vi "Sig2MS dialogPyScript.vi"(8 "error in (no error)":errorcluster) -> (0 "error out":errorcluster)   [LabVIEW 2018]
uses:
  winForms/winForms editorType.ctl
  C:/ATI_MS_InstrumentControl/dll/ScintillaNET.dll
  dll/ScintillaNET.dll
  QMH/QMH.lvclass
  Sig2MS.lvclass
  System.Windows.Forms
panel:
  in  "searchString":string
  in  "SaveScript_new":bool
  in  "open script":bool caption="OpenScript"
  in  "helper":bool caption="helpBtn"
  in  "script":refnum<k24>(container)
  in  "msgListbox":i32(listbox)
  in  "cancelBtn":bool
  in  "submitBtn":bool
  in  "stop":bool
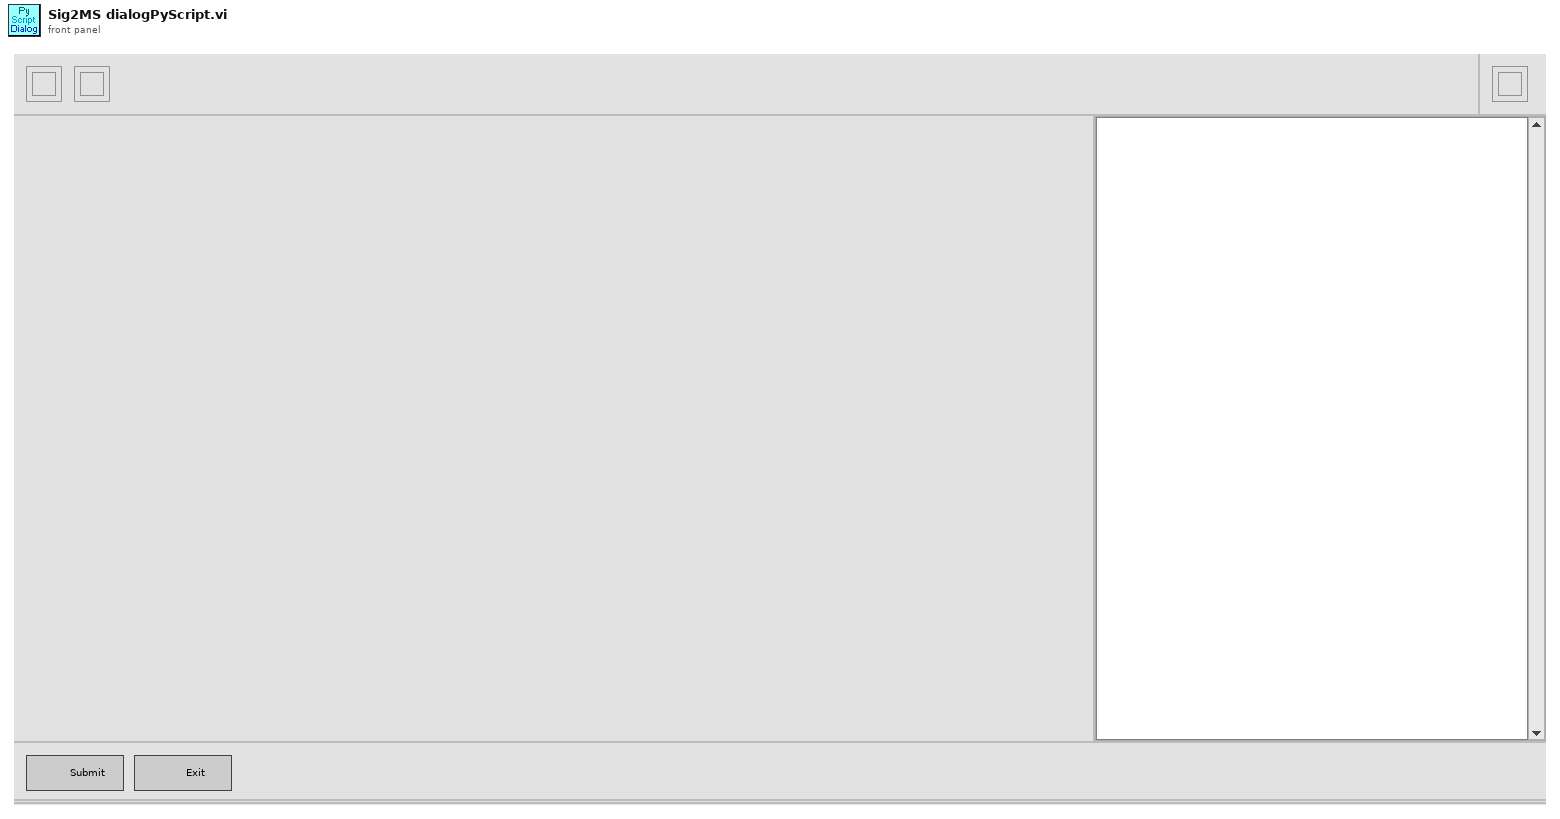
[diagram p1: front panel]
types:
  T1 = enum16{"init", "loadScript", "newScript", "runScript", "close"}
  T2 = enum8{"Enabled", "Disabled", "Disabled and Grayed Out"}
  T3 = typedef "winForms editorType.ctl" = enum16{"Recipe", "SigProc", "Editor"}
  T4 = enum16{"open", "replace", "create", "open or create", "replace or create", "replace or create with confirmation"}
  T5 = typedef "eventvkey.ctl" = enum16{"ASCII", "Enter", "Return", "Shift", "Ctrl", "Alt", "Cmd", "Opt", "Caps", "NumLock", "Clear", "Break", "Up", "Down", "Left", "Right", "Insert", "Delete", "Home", "End", "PageUp", "PageDown", "Escape", "Help", "Pause", "ScrollLock", "F1", "F2", "F3", "F4", "F5", "F6", "F7", "F8", "F9", "F10", "F11", "F12", "F13", "F14", "F15", "F16", "F17", "F18", "F19", "F20", "F21", "F22", "F23", "F24", "Play", "VolumeUp", "VolumeDown", "Mute", "Two Byte Char"}
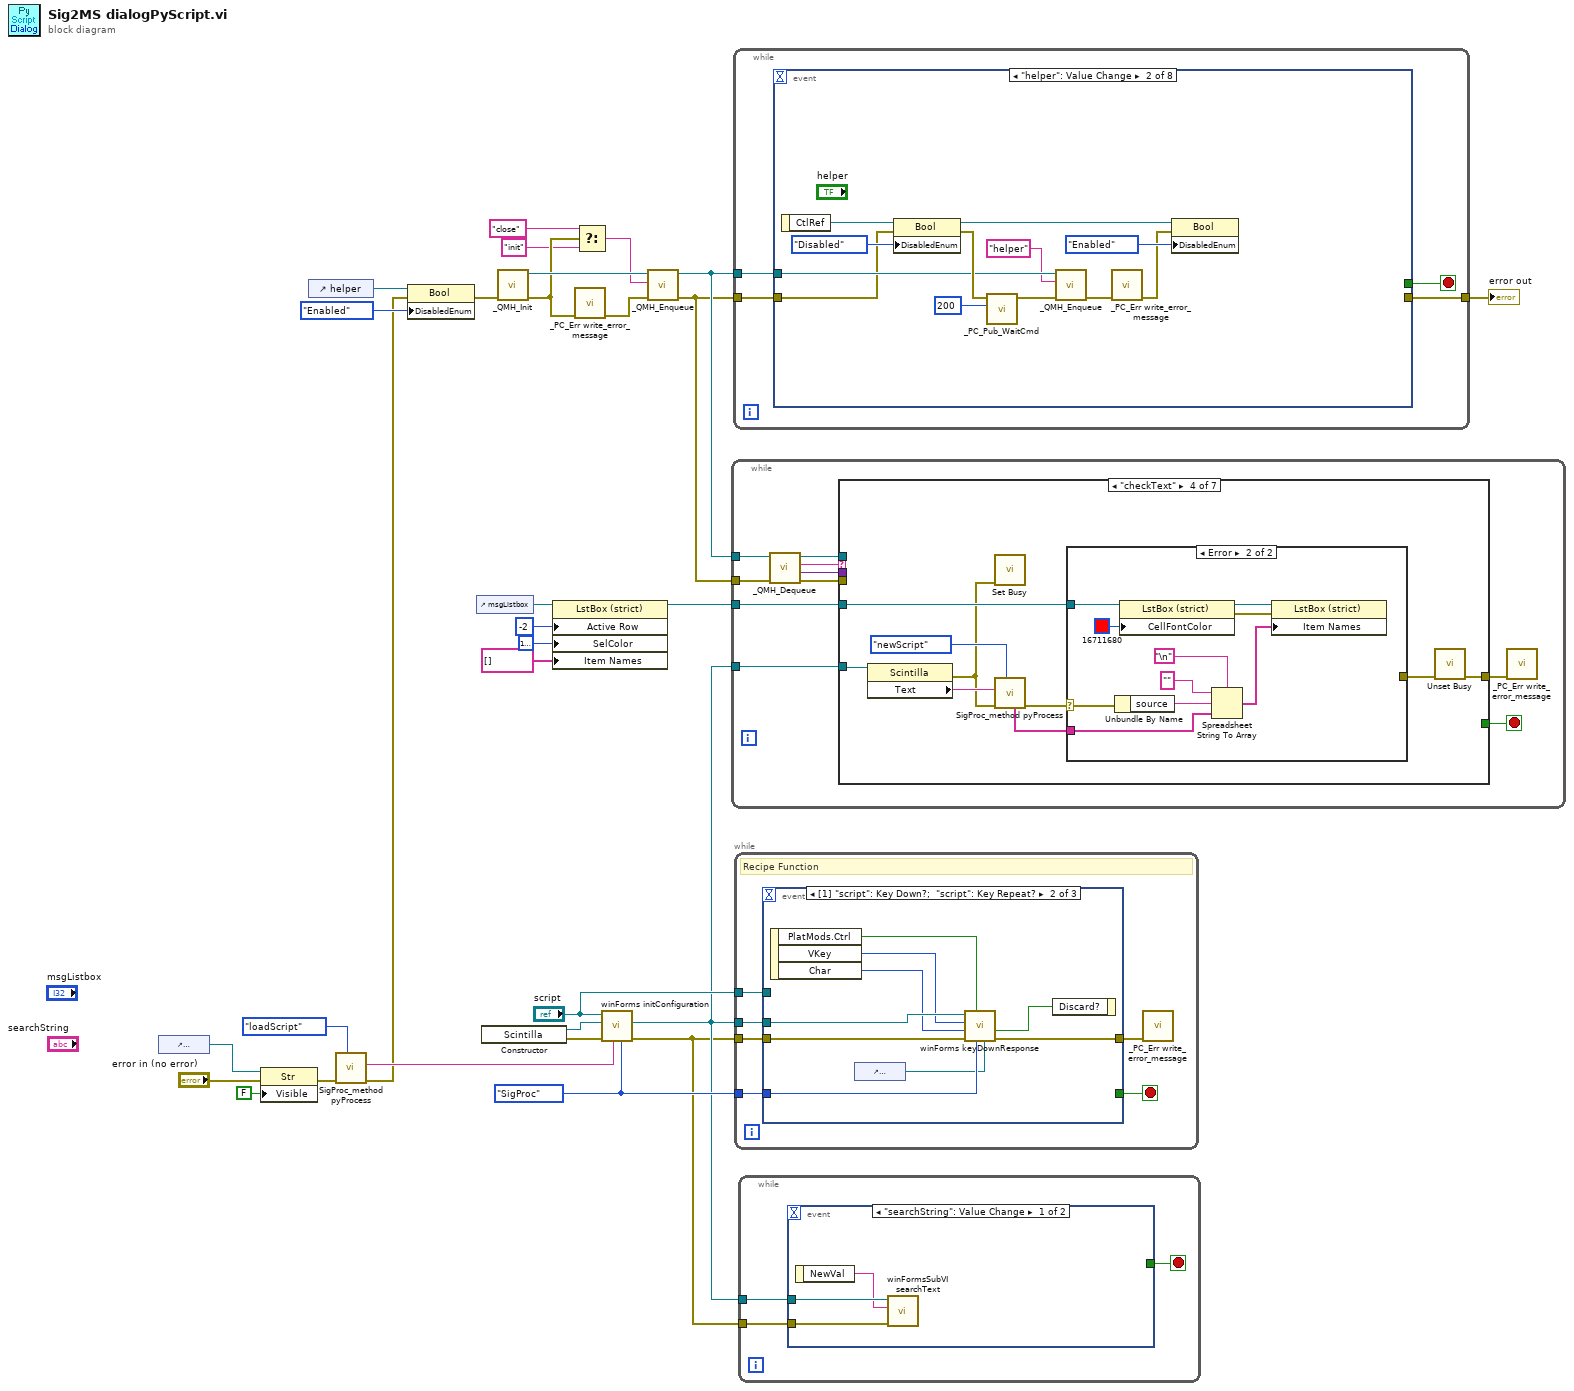
[diagram p0: block diagram]
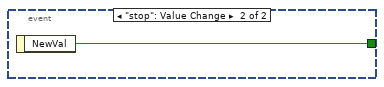
[diagram p2: hidden frame]
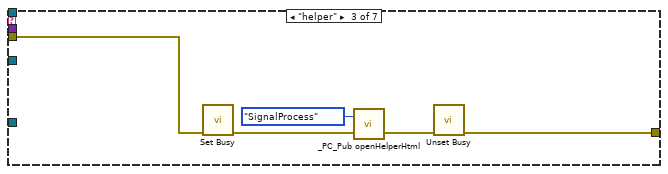
[diagram p5: hidden frame]
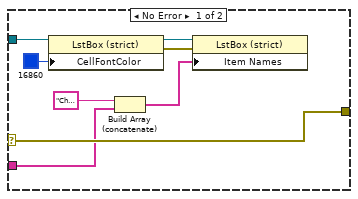
[diagram p6: hidden frame]
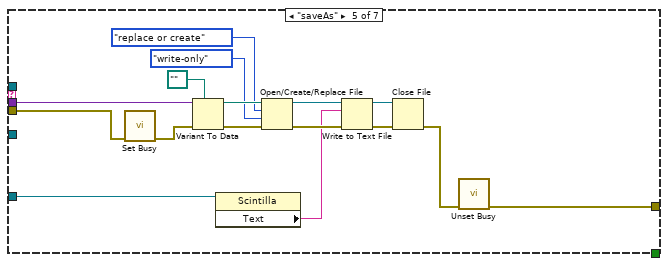
[diagram p7: hidden frame]
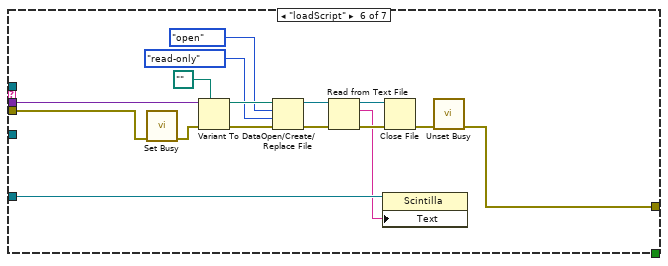
[diagram p8: hidden frame]
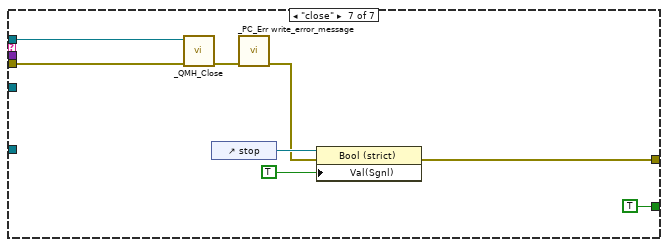
[diagram p9: hidden frame]
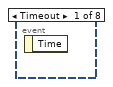
[diagram p10: hidden frame]
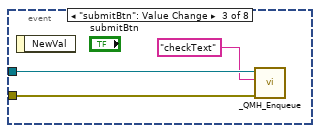
[diagram p11: hidden frame]
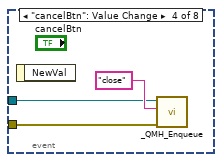
[diagram p12: hidden frame]
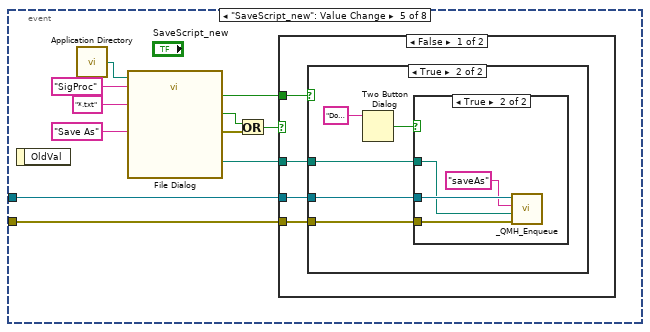
[diagram p13: hidden frame]
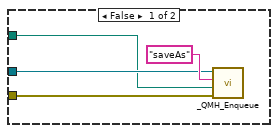
[diagram p14: hidden frame]
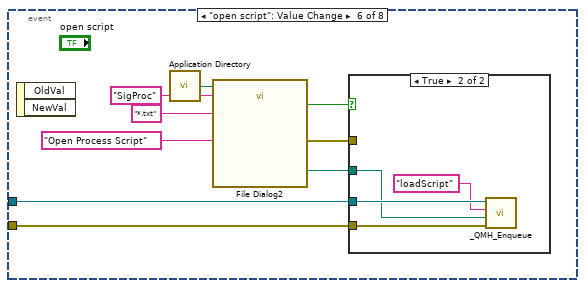
[diagram p17: hidden frame]
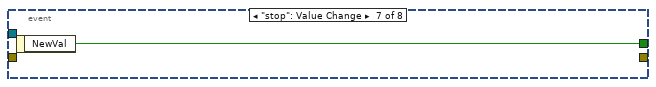
[diagram p19: hidden frame]
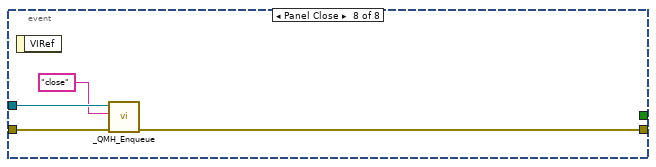
[diagram p20: hidden frame]
diagram:
  w21 = winForms_editorType."SigProc" ("editorType")
  n1 = control-ref of="searchString"() -> (w9:refnum<vi>)
  n2 = property class="Str"(reference=w9, error in="error in (no error)", "Visible"=FALSE) -> (error out=w6:errorcluster)  [unwired: 1 out]
  n3 = control-ref of="helper"() -> (w17:refnum<vi>)
  n4 = call "SigProc_method pyProcess.vi"("func"=T1."loadScript", "error in (no error)"=w6) -> ("error out"=w13:errorcluster, "pyCode"=w14:string)  [unwired: 6 in, 2 out]
  n5 = property class="Bool"(reference=w17, error in=w13, "DisabledEnum"=T2."Enabled" ("Disabled")) -> (error out=w16:errorcluster)  [unwired: 1 out]
  n6 = control-ref of="msgListbox"() -> (w1:refnum<vi>)
  n7 = constructor class="Scintilla"() -> (reference out=w30:refnum<k24>, error out=w29:errorcluster)  [unwired: 3 in, 1 out]
  n8 = call "_QMH_Init.vi"("error in (no error)"=w16) -> ("error out"=w26:errorcluster, "QMH out"=w27:refnum<class "QMH.lvclass">)  [unwired: 9 in]
  n9 = property class="LstBox (strict)"(reference=w1, "Active Row"=-2 ("Active Row:Active Row Number"), "SelColor"=u32 16777226, "Item Names"=string[] []) -> (reference out=w2:refnum<vi>)  [unwired: 1 in, 1 out]
  n10 = call "_PC_Err write_error_message.vi"("error in"=w26) -> ("error out"=w25:errorcluster)  [unwired: 10 in]
  n11 = Select(t="close", s=w26, f="init") -> (s? t:f=w24:string)
  n12 = call "winForms initConfiguration.vi"("editorType"=w21, "initText"=w14, "error in (no error)"=w29, "scintillaRefNum in"=w30, "panelRefNum"="script") -> ("error out"=w10:errorcluster, "scintillaRefNum out"=w11:refnum<k24>)  [unwired: 5 in]
  n13 = call "_QMH_Enqueue.vi"("error in (no error)"=w25, "Msg"=w24, "QMH in"=w27) -> ("error out"=w22:errorcluster, "QMH out"=w23:refnum<class "QMH.lvclass">)  [unwired: 7 in]
  n14 = while {
    tunnel: w23 -> [w40]
    tunnel: w22 -> [w39]
    tunnel: w11 -> [w34]
    tunnel: w2 -> [w31]
    stop <- w32 stop-if-true
    n15 = call "_QMH_Dequeue.vi"("error in (no error)"=w39, "QMH in"=w40) -> ("error out"=w36:errorcluster, "Data"=w37:variant, "Msg"=w38:string, "QMH out"=w35:refnum<class "QMH.lvclass">)  [unwired: 4 in, 2 out]
    n16 = case shown="\"checkText\"" w38 {
      tunnel: w37 -> [_ _ _ _ w90 w106 _]
      tunnel: w36 -> [w41 w42 w46 _ w82 w98 w113]
      tunnel: w35 -> [_ _ _ _ _ _ w114]
      tunnel: w34 -> [_ _ _ w56 w78 w94 _]
      tunnel: [w41 w42 w43 w48 w79 w95 w108] -> w33
      tunnel: [_ _ _ _ _ _ TRUE] -> w32
      tunnel: w31 -> [_ _ _ w52 _ _ _]
      frame Default {
      }
      frame "init" {
      }
      frame "helper" {
        n17 = call <vilib>:"Set Busy.vi"("error in (no error)"=w46) -> ("error out"=w45:errorcluster)  [unwired: 9 in, 1 out]
        n18 = call "_PC_Pub openHelperHtml.vi"("error in (no error)"=w45, "procType"=enum16{"none", "MSProcess", "SignalProcess"}."SignalProcess") -> ("error out"=w44:errorcluster)  [unwired: 1 out]
        n19 = call <vilib>:"Unset Busy.vi"("error in (no error)"=w44) -> ("error out"=w43:errorcluster)  [unwired: 10 in]
      }
      frame "checkText" {
        n20 = property class="Scintilla"(reference=w56) -> (error out=w51:errorcluster, "Text"=w54:string)  [unwired: 1 in, 1 out]
        n21 = call <vilib>:"Set Busy.vi"("error in (no error)"=w51) -> ()  [unwired: 9 in, 2 out]
        n22 = call "SigProc_method pyProcess.vi"("func"=T1."newScript", "error in (no error)"=w51, "newScriptCode"=w54) -> ("error out"=w53:errorcluster, "showMsg"=w50:string[])  [unwired: 5 in, 2 out]
        n23 = case shown="Error" w53 {
          selector: w53 -> [w64 w66]
          tunnel: [w64 _] -> w49
          tunnel: w52 -> [w61 w67]
          tunnel: w50 -> [w59 w65]
          frame No Error {
            n24 = property class="LstBox (strict)"(reference=w61, "CellFontColor"=u32 16860) -> (reference out=w60:refnum<vi>, error out=w62:errorcluster)  [unwired: 1 in]
            n25 = Build Array (concatenate)("Check ok...", w59) -> (w57:string[])
            n26 = property class="LstBox (strict)"(reference=w60, error in=w62, "Item Names"=w57) -> ()  [unwired: 2 out]
          }
          frame Error {
            n27 = Unbundle By Name(w66) -> ("source"=w70:string)
            n28 = property class="LstBox (strict)"(reference=w67, "CellFontColor"=u32 16711680) -> (reference out=w73:refnum<vi>, error out=w72:errorcluster)  [unwired: 1 in]
            n29 = Spreadsheet String To Array(delimiter (Tab)="\n", format string="", spreadsheet string=w70, array type (2D Dbl)=w65) -> (array=w68:string[])
            n30 = property class="LstBox (strict)"(reference=w73, error in=w72, "Item Names"=w68) -> ()  [unwired: 2 out]
          }
        }
        n31 = call <vilib>:"Unset Busy.vi"("error in (no error)"=w49) -> ("error out"=w48:errorcluster)  [unwired: 10 in]
      }
      frame "saveAs" {
        n32 = call <vilib>:"Set Busy.vi"("error in (no error)"=w82) -> ("error out"=w81:errorcluster)  [unwired: 9 in, 1 out]
        n33 = Variant To Data(error in=w81, type=path "", Variant=w90) -> (data=w88:path, error out=w87:errorcluster)
        n34 = property class="Scintilla"(reference=w78) -> ("Text"=w77:string)  [unwired: 1 in, 2 out]
        n35 = Open/Create/Replace File(file path (use dialog)=w88, error in=w87, operation (0:open)=T4."replace or create", access (0:read/write)=enum16{"read/write", "read-only", "write-only"}."write-only") -> (refnum out=w86:refnum<file>, error out=w85:errorcluster)  [unwired: 2 in, 1 out]
        n36 = Write to Text File(file (use dialog)=w86, text=w77, error in=w85) -> (refnum out=w84:refnum<file>, error out=w83:errorcluster)  [unwired: 1 in, 1 out]
        n37 = Close File(refnum=w84, error in=w83) -> (error out=w80:errorcluster)  [unwired: 1 out]
        n38 = call <vilib>:"Unset Busy.vi"("error in (no error)"=w80) -> ("error out"=w79:errorcluster)  [unwired: 10 in]
      }
      frame "loadScript" {
        n39 = call <vilib>:"Set Busy.vi"("error in (no error)"=w98) -> ("error out"=w97:errorcluster)  [unwired: 9 in, 1 out]
        n40 = Variant To Data(error in=w97, type=path "", Variant=w106) -> (data=w104:path, error out=w103:errorcluster)
        n41 = Open/Create/Replace File(file path (use dialog)=w104, error in=w103, operation (0:open)=T4."open", access (0:read/write)=enum16{"read/write", "read-only", "write-only"}."read-only") -> (refnum out=w102:refnum<file>, error out=w101:errorcluster)  [unwired: 2 in, 1 out]
        n42 = Read from Text File(file (use dialog)=w102, error in=w101) -> (refnum out=w100:refnum<file>, text=w93:string, error out=w99:errorcluster)  [unwired: 2 in, 1 out]
        n43 = property class="Scintilla"(reference=w94, "Text"=w93) -> ()  [unwired: 1 in, 2 out]
        n44 = Close File(refnum=w100, error in=w99) -> (error out=w96:errorcluster)  [unwired: 1 out]
        n45 = call <vilib>:"Unset Busy.vi"("error in (no error)"=w96) -> ("error out"=w95:errorcluster)  [unwired: 10 in]
      }
      frame "close" {
        n46 = call "_QMH_Close.vi"("error in (no error)"=w113, "QMH in"=w114) -> ("error out"=w110:errorcluster)  [unwired: 9 in]
        n47 = control-ref of="stop"() -> (w111:refnum<vi>)
        n48 = call "_PC_Err write_error_message.vi"("error in"=w110) -> ("error out"=w109:errorcluster)  [unwired: 10 in]
        n49 = property class="Bool (strict)"(reference=w111, error in=w109, "Val(Sgnl)"=TRUE ("Value (Signaling)")) -> (error out=w108:errorcluster)  [unwired: 1 out]
      }
    }
    n50 = call "_PC_Err write_error_message.vi"("error in"=w33) -> ()  [unwired: 10 in, 1 out]
  }
  n51 = while {
    tunnel: w23 -> [w117]
    tunnel: w22 -> [w116]
    tunnel: [w115] -> w12
    stop <- w118 stop-if-true
    n52 = event shown="[1] \"helper\": Value Change" {
      selector: _ -> [_ _ _ _ _ _ _ _]
      dyn-events: _ -> [_ _ _ _ _ _ _ _]
      timeout: _ -> [_ _ _ _ _ _ _ _]
      tunnel: [_ _ _ _ _ _ w178 _] -> w118
      tunnel: w117 -> [_ w123 w133 w135 w138 w166 _ w182]
      tunnel: w116 -> [_ w122 w132 w134 w137 w165 _ w181]
      tunnel: [_ _ _ _ _ _ _ w179] -> w115
      event Timeout {
        n53 = event-data() -> ()  [unwired: 1 in, 1 out]
      }
      event "helper": Value Change {
        n54 = event-data() -> ("CtlRef"=w125:refnum<vi>)  [unwired: 1 in]
        n55 = property class="Bool"(reference=w125, error in=w122, "DisabledEnum"=T2."Disabled" ("Disabled")) -> (reference out=w130:refnum<vi>, error out=w128:errorcluster)
        n56 = call "_PC_Pub_WaitCmd.vi"("milliseconds to wait"=u32 200, "error in (no error)"=w128) -> ("error out"=w121:errorcluster)  [unwired: 9 in]
        n57 = call "_QMH_Enqueue.vi"("error in (no error)"=w121, "Msg"="helper", "QMH in"=w123) -> ("error out"=w119:errorcluster)  [unwired: 7 in, 1 out]
        n58 = call "_PC_Err write_error_message.vi"("error in"=w119) -> ("error out"=w126:errorcluster)  [unwired: 10 in]
        n59 = property class="Bool"(reference=w130, error in=w126, "DisabledEnum"=T2."Enabled" ("Disabled")) -> ()  [unwired: 2 out]
      }
      event "submitBtn": Value Change {
        n60 = event-data() -> ()  [unwired: 1 in, 1 out]
        n61 = call "_QMH_Enqueue.vi"("error in (no error)"=w132, "Msg"="checkText", "QMH in"=w133) -> ()  [unwired: 7 in, 2 out]
      }
      event "cancelBtn": Value Change {
        n62 = event-data() -> ()  [unwired: 1 in, 1 out]
        n63 = call "_QMH_Enqueue.vi"("error in (no error)"=w134, "Msg"="close", "QMH in"=w135) -> ()  [unwired: 7 in, 2 out]
      }
      event "SaveScript_new": Value Change {
        n64 = event-data() -> ()  [unwired: 1 in, 1 out]
        n65 = call <vilib>:"Application Directory.vi"() -> ("Application Directory"=w147:path)
        n66 = call "File Dialog"("start path"=w147, "prompt"="Save As", "default name"="SigProc" ("pattern label"), "pattern (all files)"="*.txt") -> ("selected path"=w142:path, "exists"=w143:bool, "cancelled"=w141:bool, "error out"=w140:errorcluster)  [unwired: 8 in]
        n67 = Or(x=w141, y=w140) -> (x .or. y?=w139:bool)
        n68 = case shown="False" w139 {
          tunnel: w143 -> [w151 _]
          tunnel: w142 -> [w150 _]
          tunnel: w138 -> [w149 _]
          tunnel: w137 -> [w148 _]
          frame False {
            n69 = case shown="True" w151 {
              tunnel: w150 -> [w152 w156]
              tunnel: w149 -> [w154 w158]
              tunnel: w148 -> [w153 w157]
              frame False {
                n70 = call "_QMH_Enqueue.vi"("error in (no error)"=w153, "Data"=w152, "Msg"="saveAs", "QMH in"=w154) -> ()  [unwired: 6 in, 2 out]
              }
              frame True {
                n71 = Two Button Dialog(message="Do you want to overwrite this file?") -> (T button?=w159:bool)  [unwired: 2 in]
                n72 = case shown="True" w159 {
                  tunnel: w158 -> [_ w164]
                  tunnel: w157 -> [_ w161]
                  tunnel: w156 -> [_ w163]
                  frame False {
                  }
                  frame True {
                    n73 = call "_QMH_Enqueue.vi"("error in (no error)"=w161, "Data"=w163, "Msg"="saveAs", "QMH in"=w164) -> ()  [unwired: 6 in, 2 out]
                  }
                }
              }
            }
          }
          frame True {
          }
        }
      }
      event "open script": Value Change {
        n74 = event-data() -> ()  [unwired: 1 in, 2 out]
        n75 = call <vilib>:"Application Directory.vi"() -> ("Application Directory"=w173:path)
        n76 = call "File Dialog2"("start path"=w173, "prompt"="Open Process Script", "default name"="SigProc" ("pattern label"), "pattern (all files)"="*.txt") -> ("selected path"=w167:path, "exists"=w169:bool, "error out"=w168:errorcluster)  [unwired: 8 in, 1 out]
        n77 = case shown="True" w169 {
          tunnel: w168 -> [_ _]
          tunnel: w167 -> [_ w174]
          tunnel: w166 -> [_ w177]
          tunnel: w165 -> [_ w176]
          frame False {
          }
          frame True {
            n78 = call "_QMH_Enqueue.vi"("error in (no error)"=w176, "Data"=w174, "Msg"="loadScript", "QMH in"=w177) -> ()  [unwired: 6 in, 2 out]
          }
        }
      }
      event "stop": Value Change {
        n79 = event-data() -> ("NewVal"=w178:bool)  [unwired: 1 in]
      }
      event Panel Close {
        n80 = event-data() -> ()  [unwired: 1 in, 1 out]
        n81 = call "_QMH_Enqueue.vi"("error in (no error)"=w181, "Msg"="close", "QMH in"=w182) -> ("error out"=w179:errorcluster)  [unwired: 7 in, 1 out]
      }
    }
  }
  "error out" <- w12
  n82 = while {
    tunnel: w11 -> [w187]
    tunnel: w10 -> [w186]
    tunnel: "script" -> [w185]
    tunnel: w21 -> [w184]
    stop <- w188 stop-if-true
    # "Recipe Function"
    n83 = event shown="[1] \"script\": Key Down?;  \"script\": Key Repeat?" {
      selector: _ -> [_ _ _]
      dyn-events: _ -> [_ _ _]
      timeout: _ -> [_ _ _]
      tunnel: [_ _ w205] -> w188
      tunnel: w187 -> [_ w197 w201]
      tunnel: w186 -> [_ w196 w200]
      tunnel: w185 -> [_ _ w203]
      tunnel: w184 -> [_ w194 _]
      tunnel: [_ w193 w202] -> w183
      event Timeout {
        n84 = event-data() -> ()  [unwired: 1 in, 1 out]
      }
      event "script": Key Down?; "script": event type 3.0.x8000000b {
        n85 = event-data() -> ("PlatMods.Ctrl"=w192:bool, "VKey"=w191:T5, "Char"=w195:i16)  [unwired: 1 in]
        n86 = control-ref of="searchString"() -> (w189:refnum<vi>)
        n87 = call "winForms keyDownResponse.vi"("searchString"=w189, "editorType"=w194, "Ctrl"=w192, "error in (no error)"=w196, "Char"=w195, "VKey"=w191, "scintillaRefNum"=w197) -> ("error out"=w193:errorcluster, "Discard?"=w190:bool)  [unwired: 3 in]
        n88 = event-data("Discard?"=w190) -> ()  [unwired: 1 in, 1 out]
      }
      event "stop": Value Change {
        n89 = event-data() -> ("NewVal"=w205:bool)  [unwired: 1 in]
        n90 = invoke class="Scintilla" method="ClearAll"(reference=w201, error in=w200) -> (reference out=w198:refnum<k24>, error out=w199:errorcluster)  [unwired: 1 in, 1 out]
        n91 = Close Reference(reference=w198, error in (no error)=w199) -> (error out=w204:errorcluster)
        n92 = Close Reference(reference=w203, error in (no error)=w204) -> (error out=w202:errorcluster)
      }
    }
    n93 = call "_PC_Err write_error_message.vi"("error in"=w183) -> ()  [unwired: 10 in, 1 out]
  }
  n94 = while {
    tunnel: w11 -> [w208]
    tunnel: w10 -> [w207]
    stop <- w206 stop-if-true
    n95 = event shown="[0] \"searchString\": Value Change" {
      selector: _ -> [_ _]
      dyn-events: _ -> [_ _]
      timeout: _ -> [_ _]
      tunnel: w208 -> [w211 _]
      tunnel: w207 -> [w210 _]
      tunnel: [_ w212] -> w206
      event "searchString": Value Change {
        n96 = event-data() -> ("NewVal"=w209:string)  [unwired: 1 in]
        n97 = call "winFormsSubVI searchText.vi"("error in (no error)"=w210, "searchString"=w209, "scintillaRefNum in"=w211) -> ()  [unwired: 7 in, 2 out]
      }
      event "stop": Value Change {
        n98 = event-data() -> ("NewVal"=w212:bool)  [unwired: 1 in]
      }
    }
  }
